vi "Read.vi"(8 "error in (no error)":errorcluster, 11 "Digital Command Config in":refnum<class "Digital Command Config.lvclass">) -> (0 "error out":errorcluster, 1 "Command":bool, 2 "Channel":string, 3 "Digital Command Config out":refnum<class "Digital Command Config.lvclass">)   [LabVIEW 2020, in "VolatusSeqConfig.lvlib" / "Digital Command Config.lvclass"]
uses:
  Digital Command Config.lvclass
  Digital Command Config.lvclass/Digital Command Config.ctl
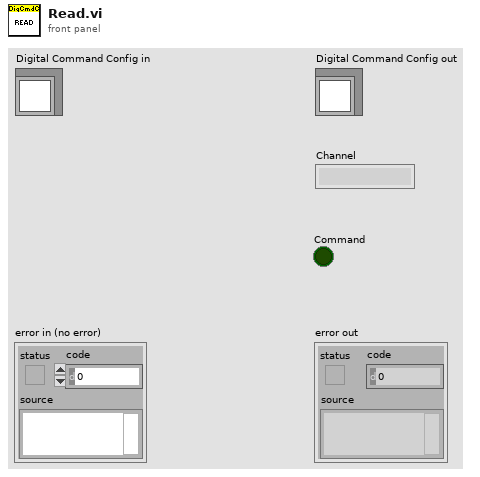
[diagram p1: front panel]
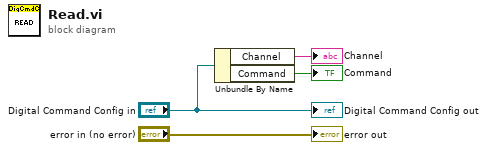
[diagram p0: block diagram]
diagram:
  n1 = Unbundle By Name("Digital Command Config in") -> ("Channel"=→"Channel":string, "Command"=→"Command":bool)
  "error out" <- "error in (no error)"
  "Digital Command Config out" <- "Digital Command Config in"
